vi "Reorder ROI data file paths in ascending filename order.vi"(6 "ROI number":i32=1 min=1, 8 "Channel A?":bool, 9 "ROI ID string":string, 10 "ROI file format version":i32, 11 "Dataset directory path":path) -> (0 "Error out":errorcluster, 3 "Reordered file paths in ascending file-name order":path[](array[path]))   [LabVIEW 2017]
panel:
  out "ROI data file paths":path[](array[path])
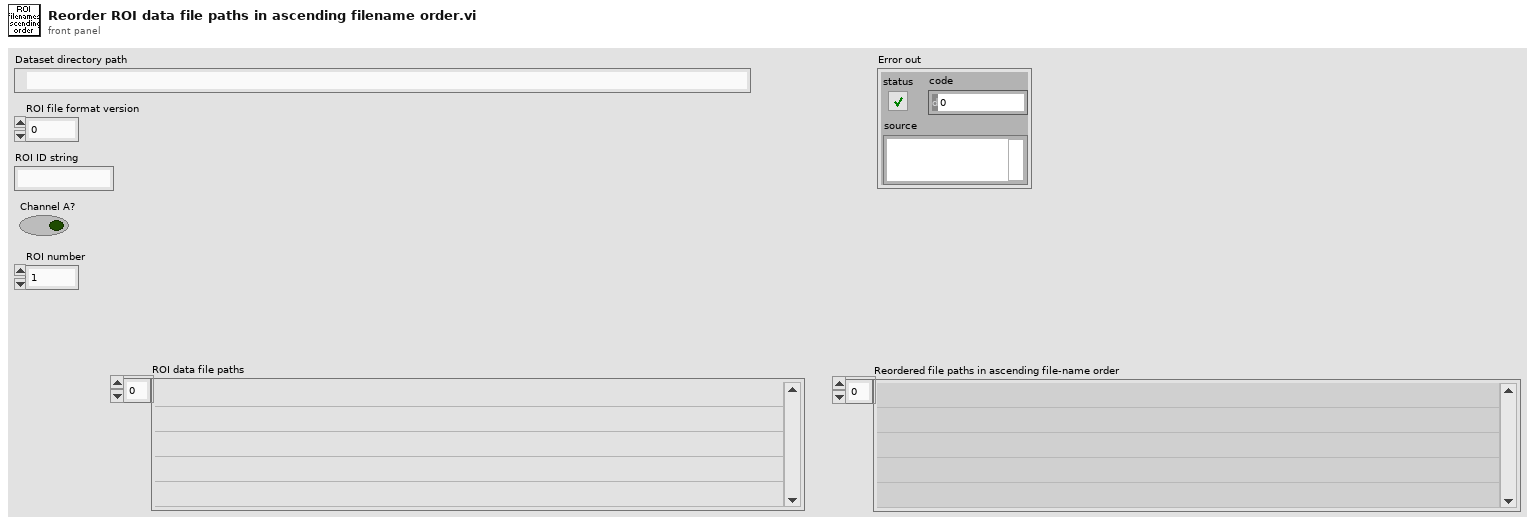
[diagram p1: front panel]
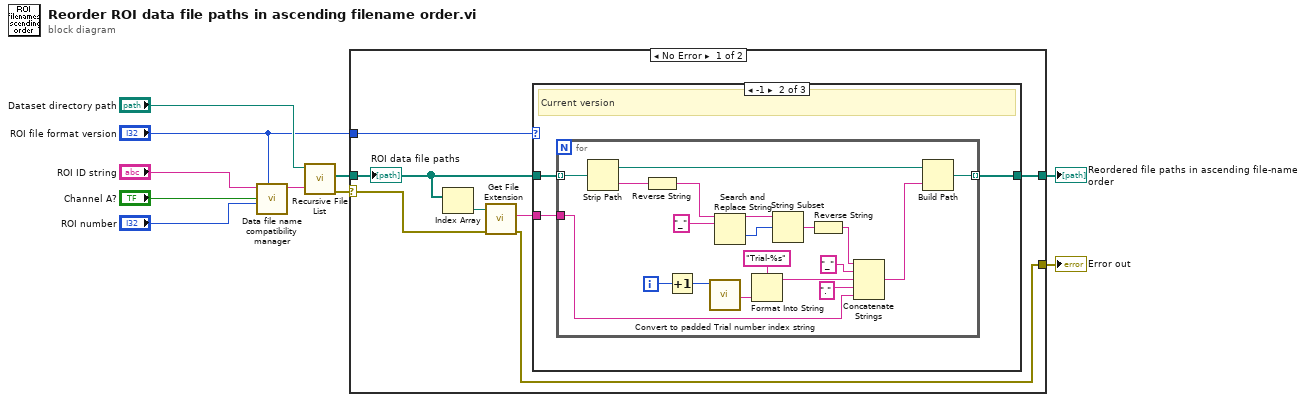
[diagram p0: block diagram]
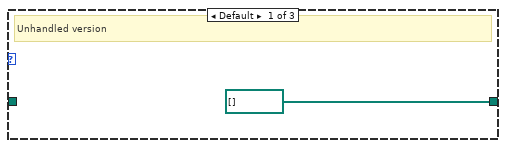
[diagram p2: hidden frame]
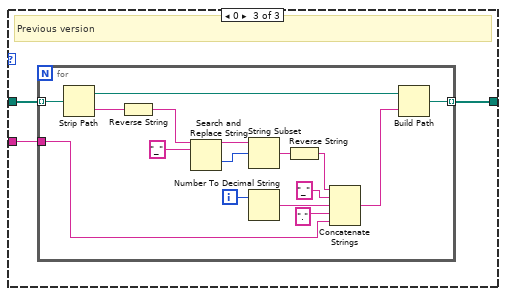
[diagram p3: hidden frame]
diagram:
  n1 = call "Data file name compatibility manager.vi"("ROI file format version"="ROI file format version", "ROI number"="ROI number", "Channel A?"="Channel A?", "ROI ID string"="ROI ID string") -> ("File name"=w6:string)  [unwired: 7 in]
  n2 = call <vilib>:"Recursive File List.vi"("pattern"=w6, "Folder Path"="Dataset directory path") -> ("error out"=w2:errorcluster, "All Files in Dir"=w4:path[])  [unwired: 5 in, 3 out]
  n3 = case shown="No Error" w2 {
    selector: w2 -> [w12 w60]
    tunnel: [w17 _] -> w10
    tunnel: w4 -> [w14 _]
    tunnel: "ROI file format version" -> [w13 _]
    tunnel: [w11 w60] -> w1
    frame No Error {
      n4 = Index Array(array=w14) -> (element=w16:path)  [unwired: 1 in]
      n5 = call <vilib>:"Get File Extension.vi"("error in (no error)"=w12, "file"=w16) -> ("error out"=w11:errorcluster, "lowercase file extension"=w15:string)  [unwired: 5 in, 3 out]
      n6 = case shown="-1" w13 {
        tunnel: [path[] [] w21 w43] -> w17
        tunnel: w15 -> [_ w20 w42]
        tunnel: w14 -> [_ w19 w41]
        frame Default {
          # "Unhandled version"
        }
        frame -1 {
          # "Current version"
          n7 = for {
            tunnel: w19 -> [w34] mode=indexing
            tunnel: [w30] -> w21 mode=indexing
            tunnel: w20 -> [w28]
            i -> [w24]
            n8 = Strip Path(path=w34) -> (stripped path=w32:path, name=w33:string)
            n9 = Reverse String(1:w33) -> (0:w40:string)
            n10 = Increment(x=w24) -> (x+1=w22:i32)
            n11 = call "Convert to padded Trial number index string.vi"("Trial number (unity-based)"=w22) -> ("Trial number string padded with zeroes"=w25:string)  [unwired: 10 in]
            n12 = Search and Replace String(input string=w40, search string="_") -> (result string=w38:string, offset past replacement=w37:i32)  [unwired: 6 in, 2 out]
            n13 = Format Into String(format string="Trial-%s" ("pattern"), w25) -> (resulting string=w23:string)  [unwired: 2 in, 1 out]
            n14 = String Subset(string=w38, offset (0)=w37) -> (substring=w36:string)  [unwired: 1 in]
            n15 = Reverse String(1:w36) -> (0:w35:string)
            n16 = Concatenate Strings(w35, "_" ("string"), w23, "." ("string"), w28) -> (w31:string)
            n17 = Build Path(base path=w32, name or relative path=w31) -> (appended path=w30:path)
          }
        }
        frame 0 {
          # "Previous version"
          n18 = for {
            tunnel: w41 -> [w51] mode=indexing
            tunnel: [w47] -> w43 mode=indexing
            tunnel: w42 -> [w45]
            i -> [w53]
            n19 = Strip Path(path=w51) -> (stripped path=w49:path, name=w50:string)
            n20 = Reverse String(1:w50) -> (0:w59:string)
            n21 = Search and Replace String(input string=w59, search string="_") -> (result string=w57:string, offset past replacement=w56:i32)  [unwired: 6 in, 2 out]
            n22 = String Subset(string=w57, offset (0)=w56) -> (substring=w54:string)  [unwired: 1 in]
            n23 = Number To Decimal String(number=w53) -> (decimal integer string=w55:string)  [unwired: 1 in]
            n24 = Reverse String(1:w54) -> (0:w52:string)
            n25 = Concatenate Strings(w52, "_" ("string"), w55, "." ("string"), w45) -> (w48:string)
            n26 = Build Path(base path=w49, name or relative path=w48) -> (appended path=w47:path)
          }
        }
      }
      "ROI data file paths" <- w14
    }
    frame Error {
    }
  }
  "Reordered file paths in ascending file-name order" <- w10
  "Error out" <- w1
